vi "register.vi"(0 "HGF_DSCMonitor":refnum<class "HGF_DSCMonitor.lvclass">, 5 "Variable URL":string, 7 "HGF_NetworkVisitor":refnum<class "HGF_NetworkVisitor.lvclass">, 9 "HGF_TriggeredEvent":refnum<class "HGF_TriggeredEvent.lvclass">, 11 "error in (no error)":errorcluster) -> (4 "dup HGF_DSCMonitor":refnum<class "HGF_DSCMonitor.lvclass">, 15 "error out":errorcluster)   [LabVIEW 2012, in "HGF_DSC.lvlib" / "HGF_DSCMonitor.lvclass"]
doc: "register a shared variable to the monitor"
uses:
  HGF_DSCMonitor.lvclass
  HGF_BaseClasses/HGF_NetworkVisitor/HGF_NetworkVisitor.lvclass
  HGF_BaseClasses/HGF_TriggeredEvent/HGF_TriggeredEvent.lvclass
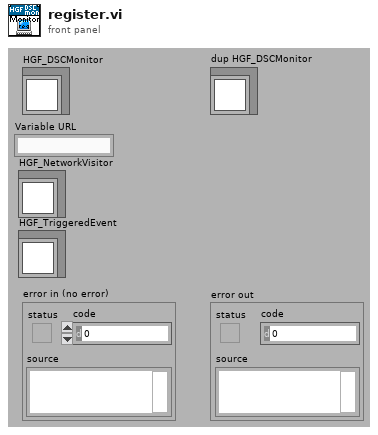
[diagram p1: front panel]
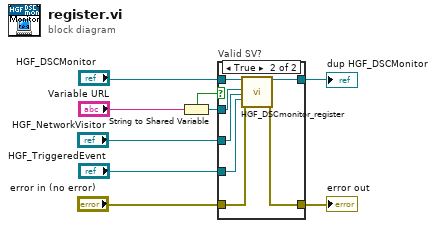
[diagram p0: block diagram]
diagram:
  n1 = String to Shared Variable(0:"Variable URL") -> (1:w3:bool, 2:w4:refnum<k21>)
  n2 = case "Valid SV?" shown="True" w3 {
    tunnel: "HGF_DSCMonitor" -> [w11 w18]
    tunnel: [w11 w17] -> w8
    tunnel: [w10 w16] -> w7
    tunnel: "HGF_NetworkVisitor" -> [_ w15]
    tunnel: w4 -> [_ w14]
    tunnel: "error in (no error)" -> [w10 w13]
    tunnel: "HGF_TriggeredEvent" -> [_ w12]
    frame False {
    }
    frame True {
      n3 = call "HGF_DSCmonitor_register.vi"("HGF_DSCMonitor in"=w18, "SV"=w14, "HGF_NetworkVisitor"=w15, "HGF_TriggeredEvent"=w12, "error in (no error)"=w13) -> ("HGF_DSCMonitor out"=w17:refnum<class "HGF_DSCMonitor.lvclass">, "error out"=w16:errorcluster)  [unwired: 13 in]
    }
  }
  "dup HGF_DSCMonitor" <- w8
  "error out" <- w7
